vi "niRFSG Configure Generation Mode.vi"(0 "instrument handle":refnum<k15>, 5 "generation mode":i32(ring)=1000 items=["CW"=1000, "Arb Waveform"=1001, "Script"=1002], 11 "error in":errorcluster {"code" format="%.0x"}) -> (4 "instrument handle out":refnum<k15>, 15 "error out":errorcluster {"code" format="%.0x"})   [LabVIEW 2014]
doc: "Configures the NI-RFSG device to generate a continuous sine tone (CW), apply I/Q (vector) modulation to the RF output signal, or generate arbitrary waveforms according to scripts. The NI-RFSG device must be in the Configuration state before you call this VI.\n\n<B>Supported Devices</B>: NI 5644R/5645R/5646R, NI 5650/5651/5652/5654/5654 with NI 5696, NI 5670/5671/5672/5673/5673E, NI 5840"
uses:
  niRFSG.dll
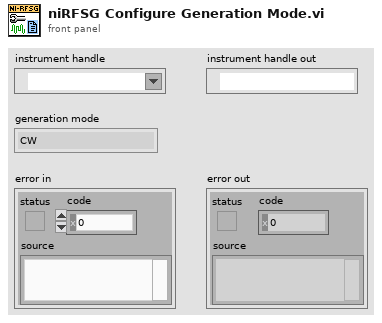
[diagram p1: front panel]
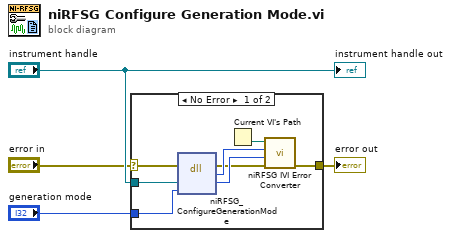
[diagram p0: block diagram]
diagram:
  n1 = case shown="No Error" "error in" {
    selector: "error in" -> [w6 w13]
    tunnel: "instrument handle" -> [w12 _]
    tunnel: [w11 w13] -> w3
    tunnel: "generation mode" -> [w7 _]
    frame No Error {
      n2 = dll-call lib="niRFSG**.*" fn="niRFSG_ConfigureGenerationMode"(error in=w6, "instrument handle"=w12, "generation mode"=w7) -> (error out=w5:errorcluster, "status"=w9:i32, "instrument handle"=w8:u32)  [unwired: 3 in, 1 out]
      n3 = Current VI's Path() -> (path=w10:path)
      n4 = call "niRFSG IVI Error Converter.vi"("error in"=w5, "instrument handle"=w8, "IVI error code"=w9, "path to VI"=w10) -> ("error out"=w11:errorcluster)  [unwired: 7 in]
    }
    frame Error {
    }
  }
  "error out" <- w3
  "instrument handle out" <- "instrument handle"
